vi "PatterMatchAlignImagesRotationMultipleFolders.vi"() -> ()   [LabVIEW 2016]
uses:
  <vilib>/Analysis/coordinate.llb/2D Cartesian Coordinate Rotation (Scalar).vi
  <vilib>/vision/NI_Vision_Development_Module.lvlib
  <vilib>/Analysis/NI_AALPro.lvlib
panel:
  in  "folder index":i32
  in  "Index Folder":i32
  in  "Angular offset":dbl
  in  "GetRotFromFileName":bool
  out "LargeSize":dbl
  in  "Shift Y":i16
  in  "Shift X":i16
  in  "Go through all":bool
  in  "RotBy":dbl
  in  "stop":bool
  out "Image":T1(plugin-control)
  in  "file index":i32
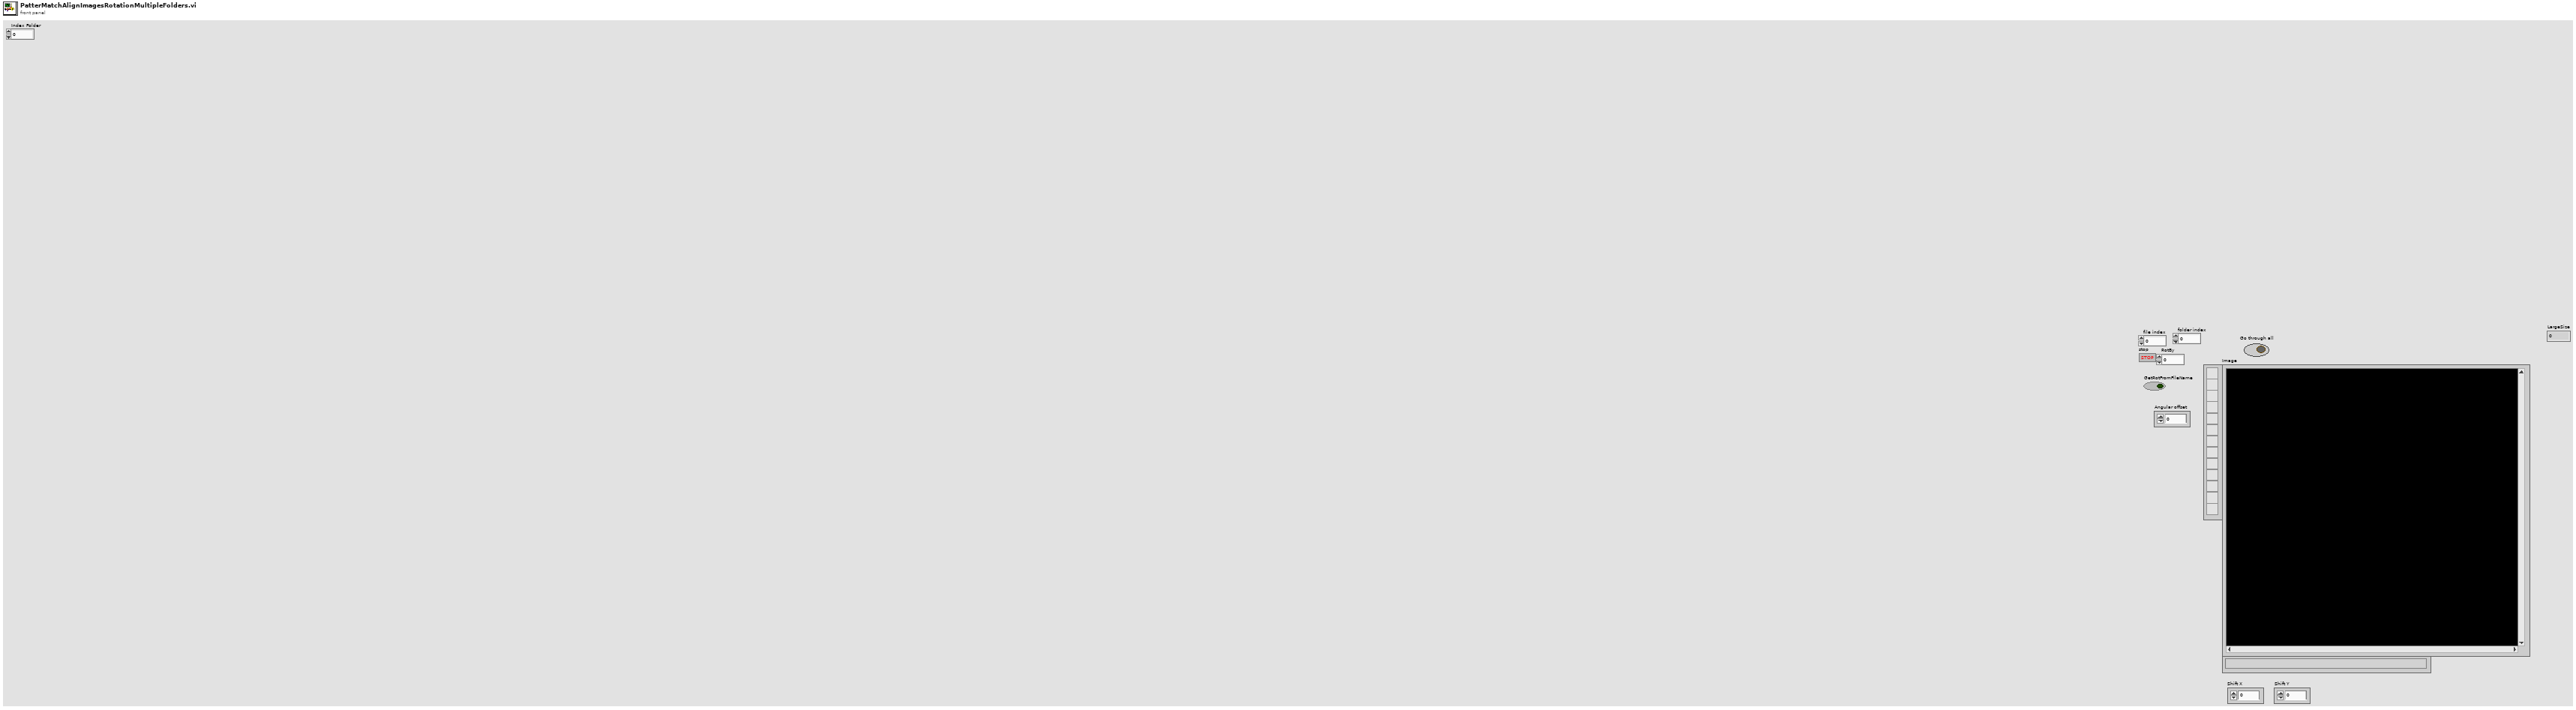
[diagram p1: front panel]
types:
  T1 = typedef "IMAQ Image.ctl" = refnum<image>
  T2 = typedef "Image Type" = u32
  T3 = cluster{"file index":i32, "Shift X":i16, "Shift Y":i16, "Angular offset":dbl, "folder index":i32}
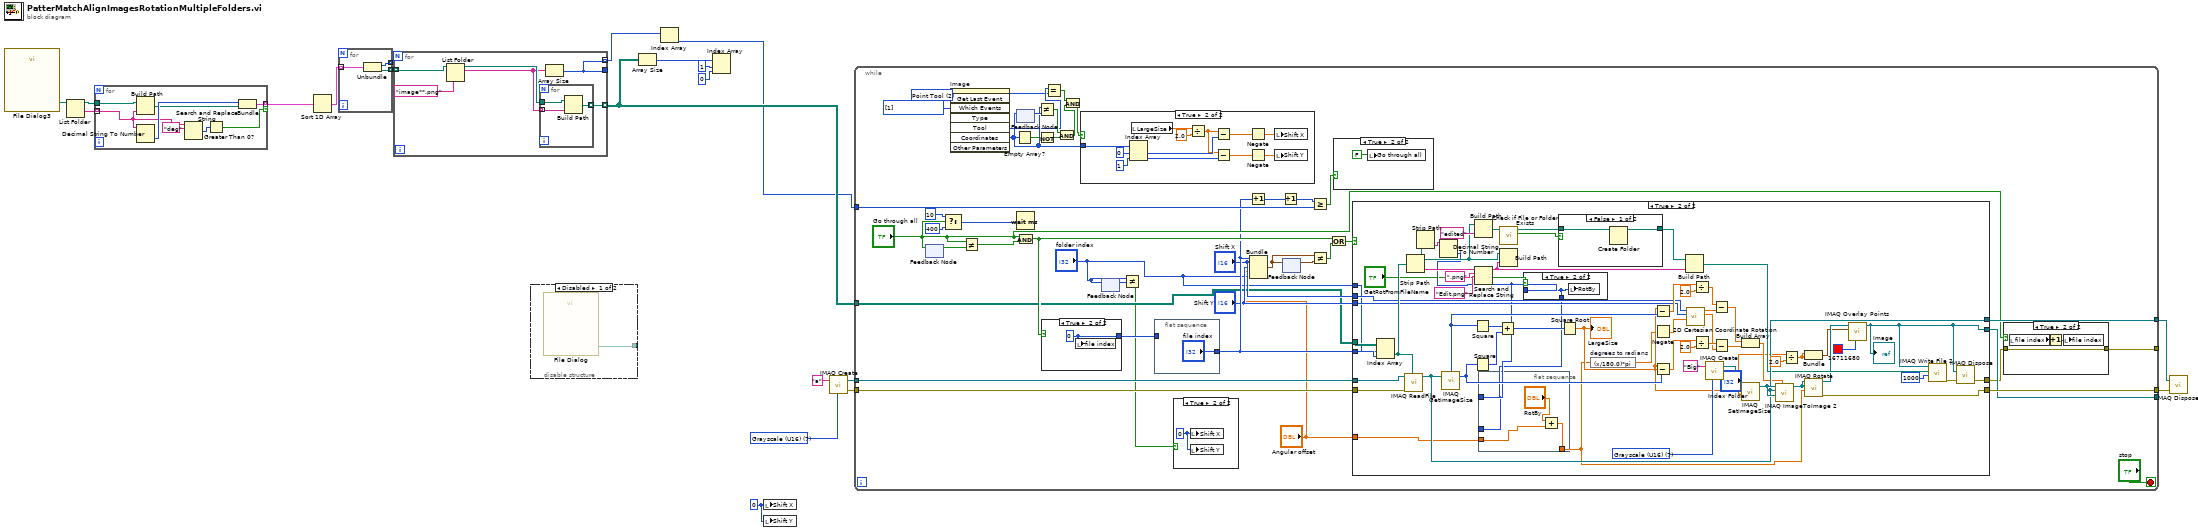
[diagram p0: block diagram]
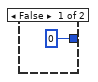
[diagram p5: hidden frame]
diagram:
  w13 = 0
  w14 = T2 7 items=["Grayscale (U8)", "Grayscale (I16)", "Grayscale (SGL)", "Complex (CSG)", "RGB (U32)", "HSL (U32)", "RGB (U64)", "Grayscale (U16)"] ("Image Type")
  n1 = call "File Dialog3"() -> ("selected path"=w12:path)  [unwired: 12 in, 3 out]
  n2 = List Folder(path=w12) -> (path out=w4:path, folder names=w5:string[])  [unwired: 3 in, 2 out]
  n3 = for {
    tunnel: w4 -> [w27]
    tunnel: [w24] -> w9 mode=indexing if=w20
    tunnel: w5 -> [w23] mode=indexing
    n4 = Build Path(base path=w27, name or relative path=w23) -> (appended path=w25:path)
    n5 = Decimal String To Number(string=w23) -> (number=w26:i32)  [unwired: 2 in, 1 out]
    n6 = Search and Replace String(input string=w23, search string="deg") -> (number of replacements=w21:i32)  [unwired: 6 in, 3 out]
    n7 = Greater Than 0?(x=w21) -> (x > 0?=w20:bool)
    n8 = Bundle(w26, "appended path"=w25) -> (w24:cluster{i32, "appended path":path})  [unwired: 1 in]
  }
  n9 = Sort 1D Array(array=w9) -> (sorted array=w8:cluster{i32, "appended path":path}[])
  n10 = for {
    tunnel: w8 -> [w30] mode=indexing
    tunnel: [w29] -> w7 mode=indexing
    tunnel: [w28] -> _ mode=indexing
    n11 = Unbundle(w30) -> (w28:i32, "appended path"=w29:path)
  }
  n12 = for {
    tunnel: [w34] -> w3 mode=indexing
    tunnel: w7 -> [w32] mode=indexing
    tunnel: [w31] -> _
    tunnel: [w31] -> w2 mode=indexing
    n13 = List Folder(path=w32, pattern="image**.png") -> (path out=w35:path, filenames=w33:string[])  [unwired: 2 in, 2 out]
    n14 = for {
      tunnel: w35 -> [w39]
      tunnel: w33 -> [w38] mode=indexing
      tunnel: [w37] -> w34 mode=indexing
      n15 = Build Path(base path=w39, name or relative path=w38) -> (appended path=w37:path)
    }
    n16 = Array Size(array=w33) -> (size(s)=w31:i32)
  }
  n17 = disable-structure shown="Disabled" {
    disable-tunnel: [w40 _] -> _
    frame Disabled {
      n18 = call "File Dialog"() -> ("selected paths"=w40:path[])  [unwired: 12 in, 3 out]
    }
    frame Enabled {
    }
  }
  n19 = Array Size(array=w3) -> (size(s)=w11:i32[])
  n20 = Index Array(array=w2) -> (element=w1:i32)  [unwired: 1 in]
  n21 = Index Array(array=w11, index #1=1 ("index"), index #2=0 ("index")) -> ()  [unwired: 2 out]
  n22 = local write "Shift X"(w13) -> ()
  n23 = local write "Shift Y"(w13) -> ()
  n24 = call "IMAQ Create"("Image Name"="a", "Image Type"=w14) -> ("New Image"=w19:T1, "error out"=w18:errorcluster)  [unwired: 3 in]
  n25 = while {
    tunnel: w19 -> [w83]
    tunnel: w18 -> [w82]
    tunnel: [w78] -> _
    tunnel: [w81] -> w17
    tunnel: [w79] -> w15
    tunnel: [w75] -> _
    tunnel: w1 -> [w74]
    tunnel: w3 -> [w44]
    stop <- "stop" stop-if-true
    w47 = 2 items=["None", "Selection Tool", "Point Tool", "Line Tool", "Rectangle Tool", "Oval Tool", "Polygon Tool", "ClosedFreehandTool", "Annulus Tool", "Rotated Rectangle Tool", "Zoom Tool", "Pan Tool", "Polyline Tool", "Freehand Tool"] ("Tool")
    w60 = i32[] [1] items=["No Event"=0, "Click Event"=1, "Draw Event"=2, "Size Event"=4, "Scroll Event"=5, "Double Click Event"=8] ("Which Events")
    n26 = feedback #1() -> (w73:bool)  [unwired: 1 in]
    n27 = feedback-in #1("Go through all") -> ()
    n28 = Select(t=u32 10, s="Go through all", f=u32 400 ("milliseconds to wait")) -> (s? t:f=w63:u32)
    n29 = invoke on="Image" class="ImageControl" method="Get Last Event"("Which Events"=w60) -> ("Tool"=w48:i32, "Coordinates"=w58:i32[])  [unwired: 7 in, 6 out]
    n30 = Not Equal?(x="Go through all", y=w73) -> (x != y?=w72:bool)
    n31 = Empty Array?(array=w58) -> (empty?=w57:bool)
    n32 = feedback #2() -> (w59:i32[])  [unwired: 1 in]
    n33 = feedback-in #2(w58) -> ()
    n34 = Wait (ms)(milliseconds to wait=w63) -> ()  [unwired: 1 out]
    n35 = And(x="Go through all", y=w72) -> (x .and. y?=w68:bool)
    n36 = Not Equal?(x=w58, y=w59) -> (x != y?=w56:bool)
    n37 = Not(x=w57) -> (.not. x?=w55:bool)
    n38 = case shown="True" w68 {
      tunnel: [0 ("index") w99] -> w71
      frame False {
      }
      frame True {
        w99 = 0 ("index")
        n39 = local write "file index"(w99) -> ()
      }
    }
    n40 = Equal?(x=w48, y=w47) -> (x = y?=w49:bool)
    n41 = And(x=w56, y=w55) -> (x .and. y?=w50:bool)
    n42 = And(x=w49, y=w50) -> (x .and. y?=w46:bool)
    n43 = case shown="True" w46 {
      tunnel: w58 -> [_ w94]
      frame False {
      }
      frame True {
        n44 = Index Array(array=w94, index #1=0 ("index"), index #2=1 ("index")) -> (element #1=w91:i32, element #2=w89:i32)
        n45 = local read "LargeSize"() -> (w96:dbl)
        n46 = Divide(x=w96, y=2.0) -> (x/y=w90:dbl)
        n47 = Subtract(x=w90, y=w91) -> (x-y=w88:dbl)
        n48 = Subtract(x=w90, y=w89) -> (x-y=w86:dbl)
        n49 = Negate(x=w88) -> (-x=w87:dbl)
        n50 = Negate(x=w86) -> (-x=w85:dbl)
        n51 = local write "Shift X"(w87) -> ()
        n52 = local write "Shift Y"(w85) -> ()
      }
    }
    n53 = feedback #3() -> (w43:i32)  [unwired: 1 in]
    n54 = feedback-in #3("folder index") -> ()
    n55 = Not Equal?(x="folder index", y=w43) -> (x != y?=w41:bool)
    n56 = flat-sequence {
      tunnel: ["file index"] -> w54
      tunnel: w71 -> [_]
      frame #0 {
      }
    }
    n57 = case shown="True" w41 {
      frame False {
      }
      frame True {
        w84 = 0
        n58 = local write "Shift X"(w84) -> ()
        n59 = local write "Shift Y"(w84) -> ()
      }
    }
    n60 = Increment(x=w54) -> (x+1=w62:i32)
    n61 = Bundle("file index"=w54, "Shift X"="Shift X", "Shift Y"="Shift Y", "Angular offset"="Angular offset", "folder index"="folder index") -> (w51:T3)  [unwired: 1 in]
    n62 = Increment(x=w62) -> (x+1=w61:i32)
    n63 = feedback-in #4(w51) -> ()
    n64 = feedback #4() -> (w77:T3)  [unwired: 1 in]
    n65 = Greater Or Equal?(x=w61, y=w74) -> (x >= y?=w67:bool)
    n66 = Not Equal?(x=w51, y=w77) -> (x != y?=w69:bool)
    n67 = Or(x=w68, y=w69) -> (x .or. y?=w70:bool)
    n68 = case shown="True" w67 {
      frame False {
      }
      frame True {
        n69 = local write "Go through all"(FALSE ("Go through all")) -> ()
      }
    }
    n70 = case shown="True" w70 {
      tunnel: w83 -> [w106 w166]
      tunnel: w82 -> [w105 w165]
      tunnel: w54 -> [_ w108]
      tunnel: [w105 w163] -> w81
      tunnel: [w106 w154] -> w79
      tunnel: [w106 w130] -> w78
      tunnel: [w105 w150] -> w76
      tunnel: "Shift X" -> [_ w122]
      tunnel: "Shift Y" -> [_ w121]
      tunnel: "Angular offset" -> [_ w110]
      tunnel: "folder index" -> [_ w107]
      tunnel: w44 -> [_ w109]
      frame False {
      }
      frame True {
        w147 = T2 7 items=["Grayscale (U8)", "Grayscale (I16)", "Grayscale (SGL)", "Complex (CSG)", "RGB (U32)", "HSL (U32)", "RGB (U64)", "Grayscale (U16)"] ("Image Type")
        n71 = Index Array(array=w109, index (row)=w107, index (col)=w108) -> (element=w164:path)
        n72 = call "IMAQ ReadFile"("File Path"=w164, "error in (no error)"=w165, "Image"=w166) -> ("Image Out"=w154:T1)  [unwired: 4 in, 4 out]
        n73 = Strip Path(path=w164) -> (stripped path=w116:path, name=w162:string)
        n74 = Strip Path(path=w116) -> (name=w115:string)  [unwired: 1 out]
        n75 = Decimal String To Number(string=w115) -> (number=w114:i32)  [unwired: 2 in, 1 out]
        n76 = call "IMAQ GetImageSize"("Image"=w154) -> ("Y Resolution"=w149:i32, "X Resolution"=w153:i32)  [unwired: 3 in, 1 out]
        n77 = Square(x=w153) -> (x^2=w158:i32)
        n78 = Square(x=w149) -> (x^2=w159:i32)
        n79 = Build Path(base path=w116, name or relative path="edited") -> (appended path=w137:path)
        n80 = Search and Replace String(input string=w162, search string=".png", replace string="Edit.png" ("replace string (\"\")")) -> (result string=w133:string)  [unwired: 5 in, 3 out]
        n81 = flat-sequence {
          tunnel: [w170] -> w112
          tunnel: w114 -> [_]
          tunnel: w111 -> [_]
          tunnel: w110 -> [w169]
          frame #0 {
            n82 = Add(x="RotBy", y=w169) -> (x+y=w170:dbl)
          }
        }
        n83 = Add(x=w158, y=w159) -> (x+y=w157:i32)
        n84 = call <vilib>:"Check if File or Folder Exists.vi"("path"=w137) -> ("file or folder exists?"=w136:bool, "dup path"=w135:path)  [unwired: 8 in, 1 out]
        n85 = Build Path(base path=w116, name or relative path=w133) -> ()  [unwired: 1 out]
        n86 = case shown="True" "GetRotFromFileName" {
          tunnel: w114 -> [w167 w168]
          tunnel: [w167 w168] -> w111
          frame False {
          }
          frame True {
            n87 = local write "RotBy"(w168) -> ()
          }
        }
        n88 = case shown="False" w136 {
          tunnel: w135 -> [w173 w174]
          tunnel: [w172 w174] -> w134
          frame False {
            n89 = Create Folder(path (use dialog)=w173) -> (created path=w172:path)  [unwired: 2 in, 2 out]
          }
          frame True {
          }
        }
        n90 = Square Root(x=w157) -> (sqrt(x)=w124:dbl)
        "LargeSize" <- w124
        n91 = expression code="(x/180.0)*pi" "degrees to radians"(w112) -> (w120:dbl)
        n92 = Subtract(x=w124, y=w153) -> (x-y=w144:dbl)
        n93 = Negate(x=w120) -> (-x=w119:dbl)
        n94 = Subtract(x=w124, y=w149) -> (x-y=w142:dbl)
        n95 = Build Path(base path=w134, name or relative path=w133) -> (appended path=w132:path)
        n96 = call-poly <vilib>:"2D Cartesian Coordinate Rotation.vi"("theta"=w119, "y"=w121, "x"=w122) -> ("y out"=w117:dbl, "x out"=w118:dbl)  [unwired: 6 in, 1 out]
        n97 = Divide(x=w144, y=2.0) -> (x/y=w129:dbl)
        n98 = Divide(x=w142, y=2.0) -> (x/y=w128:dbl)
        n99 = call "IMAQ Create"("Image Name"="Big", "Image Type"=w147) -> ("New Image"=w151:T1)  [unwired: 3 in, 1 out]
        n100 = Subtract(x=w129, y=w118) -> (x-y=w141:dbl)
        n101 = Subtract(x=w128, y=w117) -> (x-y=w140:dbl)
        n102 = Build Array(w141, w140) -> (w139:dbl[])
        n103 = call "IMAQ SetImageSize"("Y Resolution"=w124, "X Resolution"=w124, "Image"=w151) -> ("Image Out"=w156:T1)  [unwired: 2 in, 1 out]
        n104 = call "IMAQ ImageToImage 2"("Offset Left/Top"=w139, "Image Dst"=w156, "Image Src (Small)"=w154, "Image Src (Large)"=w156) -> ("Image Dst Out"=w155:T1)  [unwired: 6 in, 1 out]
        n105 = Divide(x=w124, y=2.0) -> (x/y=w123:dbl)
        n106 = Bundle(w123, w123) -> (w127:cluster{dbl, dbl})  [unwired: 1 in]
        n107 = call "IMAQ Rotate"("Angle (degrees)"=w112, "Image Dst"=w155, "Image Src"=w155) -> ("error out"=w163:errorcluster, "Image Dst Out"=w131:T1)  [unwired: 7 in]
        n108 = call "IMAQ Overlay Points"("Color"=u32 16711680, "Point"=w127, "Image"=w131) -> ("Image Out"=w130:T1)  [unwired: 7 in, 1 out]
        "Image" <- w130
        n109 = call-poly "IMAQ Write File 2"("Image Quality"=u32 1000, "File Path"=w132, "Image"=w130) -> ("error out"=w146:errorcluster)  [unwired: 7 in, 1 out]
        n110 = call "IMAQ Dispose"("Image"=w130, "error in (no error)"=w146) -> ("error out"=w150:errorcluster)  [unwired: 4 in]
      }
    }
    n111 = case shown="True" "Go through all" {
      tunnel: w76 -> [w101 w104]
      tunnel: [w101 w104] -> w75
      frame False {
      }
      frame True {
        n112 = local read "file index"() -> (w103:i32)
        n113 = Increment(x=w103) -> (x+1=w102:i32)
        n114 = local write "file index"(w102) -> ()
      }
    }
  }
  n115 = call "IMAQ Dispose"("Image"=w15, "error in (no error)"=w17) -> ()  [unwired: 4 in, 1 out]
